vi "Comments.Create Lockin AO Description.vi"(7 "error in (no error)":errorcluster, 10 "Control Experiment":refnum<class "Control Experiment.lvclass">) -> (0 "error out":errorcluster, 2 "AO Section":string, 3 "Control Experiment out":refnum<class "Control Experiment.lvclass">)   [LabVIEW 2016, in "Control Experiment.lvclass"]
uses:
  Control Experiment.lvclass
  Control Experiment.lvclass/Control Experiment.ctl
  <userlib>/LevyLab/Lockin-Multichannel/Instrument.Lockin/Instrument.Lockin.lvclass
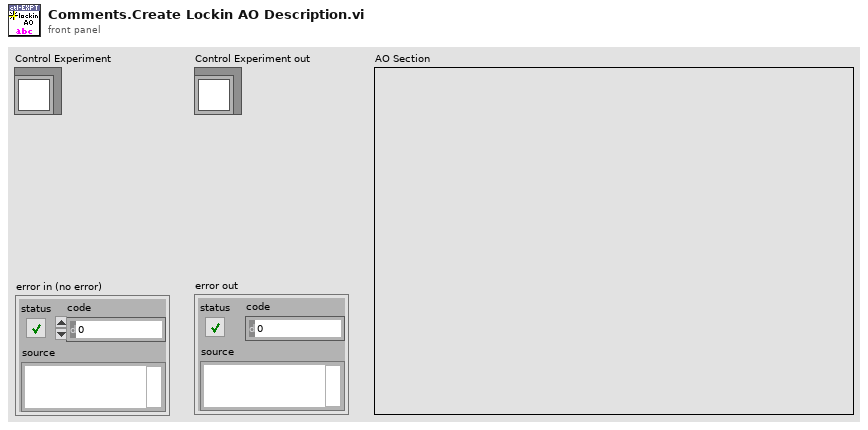
[diagram p1: front panel]
types:
  T1 = typedef "Instrument.Lockin.lvclass/AO-cluster.ctl" = cluster{"AO Amp (V)":T2, "AO DC (V)":T3, "AO f (Hz)":T4, "AO Phase (°)":T5, "Function":T6, "I+":bool[], "Sweeping":bool[]}
  T2 = typedef "Instrument.Lockin.lvclass/AO_Amp-array.ctl" = dbl[]
  T3 = typedef "Instrument.Lockin.lvclass/AO_DC-array.ctl" = dbl[]
  T4 = typedef "Instrument.Lockin.lvclass/AO_f-array.ctl" = dbl[]
  T5 = typedef "Instrument.Lockin.lvclass/AO_phi-array.ctl" = dbl[]
  T6 = typedef "Instrument.Lockin.lvclass/Function-array.ctl" = T7[]
  T7 = typedef "Instrument.Lockin.lvclass/Function-enum.ctl" = enum16{"Sine", "Triangle", "Square", "Sawtooth"}
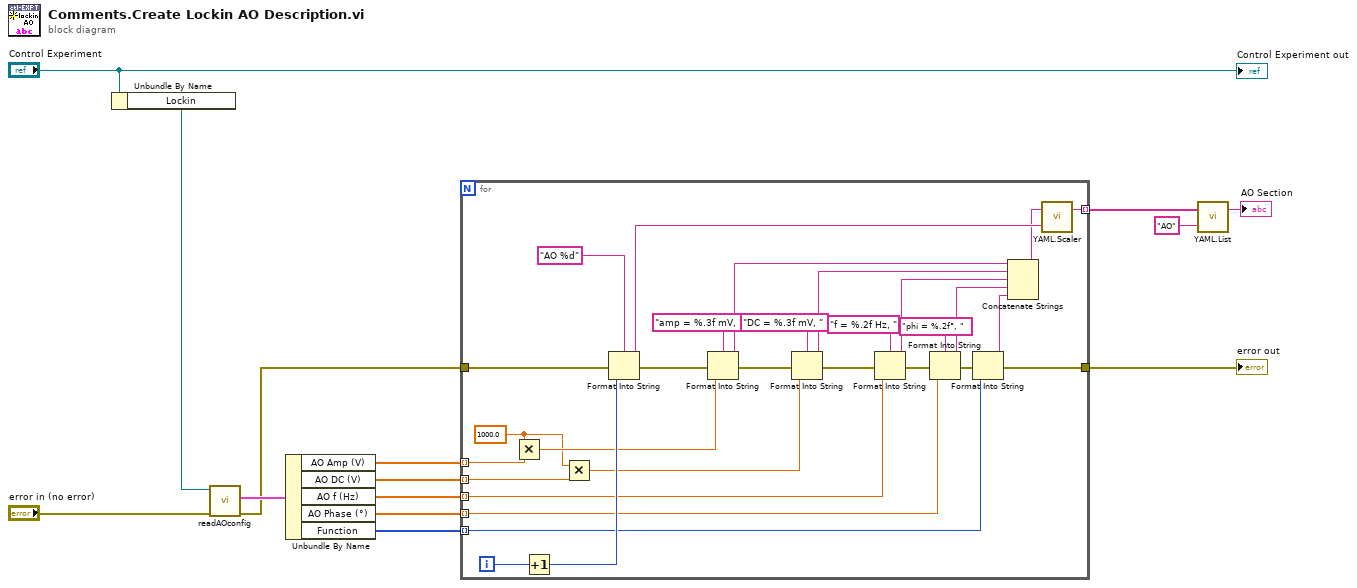
[diagram p0: block diagram]
diagram:
  n1 = Unbundle By Name("Control Experiment") -> ("Lockin"=w2:refnum<class "Instrument.Lockin.lvclass">)
  n2 = call <userlib>:"readAOconfig.vi"("error in (no error)"="error in (no error)", "Instrument.Lockin in"=w2) -> ("error out"=w3:errorcluster, "AOconfig"=w4:T1)  [unwired: 7 in, 1 out]
  n3 = Unbundle By Name(w4) -> ("AO Amp (V)"=w10:T2, "AO DC (V)"=w9:T3, "AO f (Hz)"=w8:T4, "AO Phase (°)"=w7:T5, "Function"=w6:T6)
  n4 = for {
    tunnel: w10 -> [w21] mode=indexing
    tunnel: w9 -> [w22] mode=indexing
    tunnel: w8 -> [w29] mode=indexing
    tunnel: w7 -> [w27] mode=indexing
    tunnel: w6 -> [w28] mode=indexing
    tunnel: [w15] -> w5 mode=indexing
    tunnel: w3 -> [w44]
    tunnel: [w39] -> w14
    i -> [w37]
    w18 = 1000.0 ("x")
    n5 = Multiply(x=w18, y=w21) -> (x*y=w19:dbl)
    n6 = Increment(x=w37) -> (x+1=w32:i32)
    n7 = Multiply(x=w18, y=w22) -> (x*y=w20:dbl)
    n8 = Format Into String(format string="AO %d", error in=w44, w32) -> (resulting string=w17:string, error out=w43:errorcluster)  [unwired: 1 in]
    n9 = Format Into String(format string="amp = %.3f mV, ", error in=w43, w19) -> (resulting string=w34:string, error out=w38:errorcluster)  [unwired: 1 in]
    n10 = Format Into String(format string="DC = %.3f mV, ", error in=w38, w20) -> (resulting string=w31:string, error out=w42:errorcluster)  [unwired: 1 in]
    n11 = Format Into String(format string="f = %.2f Hz, ", error in=w42, w29) -> (resulting string=w26:string, error out=w41:errorcluster)  [unwired: 1 in]
    n12 = Format Into String(format string="phi = %.2f°, ", error in=w41, w27) -> (resulting string=w24:string, error out=w40:errorcluster)  [unwired: 1 in]
    n13 = Format Into String(error in=w40, w28) -> (resulting string=w23:string, error out=w39:errorcluster)  [unwired: 2 in]
    n14 = Concatenate Strings(w34, w31, w26, w24, w23) -> (w16:string)
    n15 = call "YAML.Scaler.vi"("Key"=w17, "Scaler"=w16) -> ("Output"=w15:string)  [unwired: 1 in]
  }
  "error out" <- w14
  n16 = call "YAML.List.vi"("Key"="AO" ("string"), "lines"=w5) -> ("Output"=→"AO Section":string)  [unwired: 1 in]
  "Control Experiment out" <- "Control Experiment"
